vi "Demo - Object Data.vi"() -> ()   [LabVIEW 2021]
uses:
  DoublyNode/DoublyNode.lvclass
  CustomeData/CustomeData.lvclass
  DoublyLinkedList/DoublyLinkedList.lvclass
  IDoublyNode/IDoublyNode.lvclass
panel:
  out "previous":refnum<data-value>
  out "error out":errorcluster
  out "data":i32[](array[numeric])
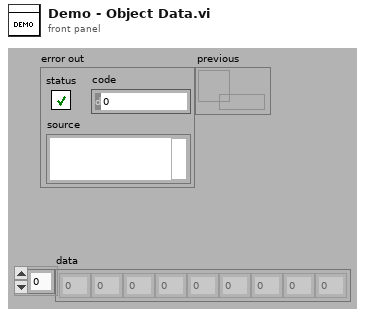
[diagram p1: front panel]
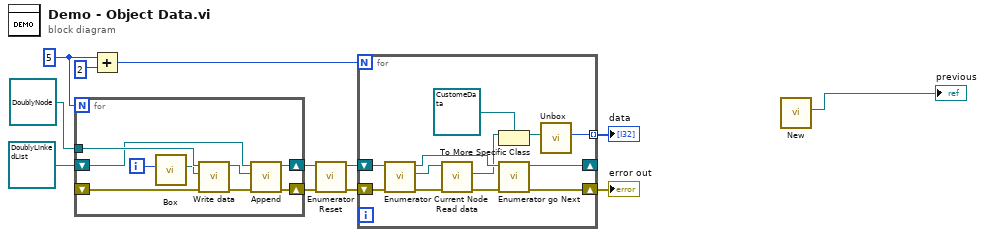
[diagram p0: block diagram]
diagram:
  w10 = 5
  n1 = for {
    N: w10 -> [_]
    tunnel: refnum<class "DoublyNode.lvclass"> refnum ("Node.lvclass") -> [w21]
    shift-right: [w13] -> w7
    shift-left: refnum<class "DoublyLinkedList.lvclass"> refnum ("DoublyLinkedList.lvclass") -> [w17]
    shift-right: [w14] -> w6
    shift-left: _ -> [w20]
    i -> [w19]
    n2 = call "Box.vi"("data"=w19) -> ("CustomeData out"=w18:refnum<class "CustomeData.lvclass">)  [unwired: 10 in]
    n3 = call-dynamic "Write data.vi"("error in (no error)"=w20, "data"=w18, "Node in"=w21) -> ("error out"=w15:errorcluster, "Node out"=w16:refnum<class "DoublyNode.lvclass">)  [unwired: 7 in]
    n4 = call-dynamic "Append.vi"("error in (no error)"=w15, "list node"=w16, "List in"=w17) -> ("error out"=w14:errorcluster, "List out"=w13:refnum<class "DoublyLinkedList.lvclass">)  [unwired: 7 in]
  }
  n5 = Add(x=w10, y=2) -> (x+y=w8:i32)
  n6 = call-dynamic "Enumerator Reset.vi"("error in (no error)"=w6, "List in"=w7) -> ("error out"=w5:errorcluster, "List out"=w4:refnum<class "DoublyLinkedList.lvclass">)  [unwired: 8 in]
  n7 = for {
    N: w8 -> [_]
    shift-right: [w33] -> _
    shift-left: w4 -> [w27]
    shift-right: [w32] -> w11
    shift-left: w5 -> [w26]
    tunnel: [w25] -> w3 mode=indexing
    n8 = call-dynamic "Enumerator Current Node.vi"("error in (no error)"=w26, "List in"=w27) -> ("error out"=w28:errorcluster, "Node"=w29:refnum<class "DoublyNode.lvclass">, "List out"=w30:refnum<class "DoublyLinkedList.lvclass">)  [unwired: 7 in]
    n9 = call-dynamic "Read data.vi"("error in (no error)"=w28, "Node in"=w29) -> ("error out"=w31:errorcluster, "data"=w23:refnum<class>)  [unwired: 7 in, 1 out]
    n10 = To More Specific Class(target class=refnum<class "CustomeData.lvclass"> refnum ("CustomeData.lvclass"), reference=w23) -> (specific class reference=w22:refnum<class "CustomeData.lvclass">)  [unwired: 1 in, 1 out]
    n11 = call-dynamic "Enumerator go Next.vi"("error in (no error)"=w31, "List in"=w30) -> ("error out"=w32:errorcluster, "List out"=w33:refnum<class "DoublyLinkedList.lvclass">)  [unwired: 8 in]
    n12 = call "Unbox.vi"("CustomeData in"=w22) -> ("data"=w25:i32)  [unwired: 10 in]
  }
  "data" <- w3
  "error out" <- w11
  n13 = call-dynamic "New.vi"() -> ("data value reference"=→"previous":refnum<data-value>)  [unwired: 9 in, 2 out]
